vi "Thermocouple - SW-Timed Input.vi"() -> ()   [LabVIEW 2022 SP3]
doc: "This example demonstrates how to continuously acquire thermocouple measurements using a DAQmx device.\n\nFor instructions on how to connect your signals to the DAQ device, refer to your device documentation."
uses:
  <vilib>/Utility/error.llb/DialogType.ctl
  <vilib>/DAQmx/read.llb/DAQmx Read (Analog 1D Wfm NChan 1Samp).vi
  <vilib>/DAQmx/create/channels.llb/DAQmx Create Channel (AI-Temperature-Thermocouple).vi
  <vilib>/DAQmx/miscellaneous.llb/DAQmx Fill In Error Info.vi
  <resource>/objmgr/daqmx.rc
panel:
  in  "Auto Zero Mode":i32(ring)=10230 items=["None"=10230, "Once"=10244, "Every Sample"=10164]
  in  "CJC Channel":refnum<k21>
  in  "CJC Value":dbl=25.0 format="%0.2f"
  in  "CJC Source":i32(ring)=10116 items=["Built-In"=10200, "Constant Value"=10116, "Channel"=10113]
  in  "Thermocouple Type":i32(ring)=10072 items=["J"=10072, "K"=10073, "N"=10077, "R"=10082, "S"=10085, "T"=10086, "B"=10047, "E"=10055]
  in  "Units":i32(ring)=10143 items=["Deg C"=10143, "Deg F"=10144, "Kelvins"=10325, "Deg R"=10145, "From Custom Scale"=10065]
  in  "Loop Time (ms)":u32=100
  in  "Stop":bool
  in  "Max Temperature":dbl=100.0
  in  "Min Temperature":dbl
  in  "Physical Channel":tag="Dev1/ai0"
  out "Waveform Chart":waveform(dbl)[](graph)
  # "Acquired Data"
  # "Channel Settings"
  # "Timing Settings"
  # "Auto Zero Settings"
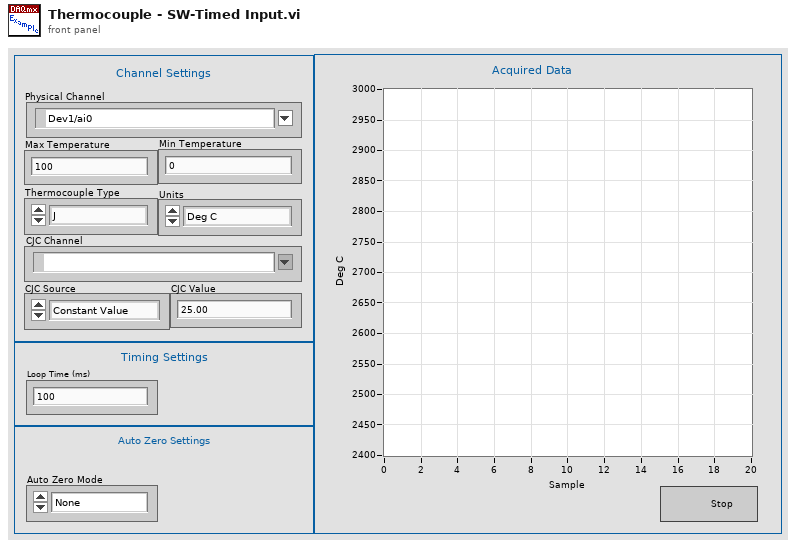
[diagram p1: front panel]
types:
  T1 = typedef "DialogType.ctl" = u16
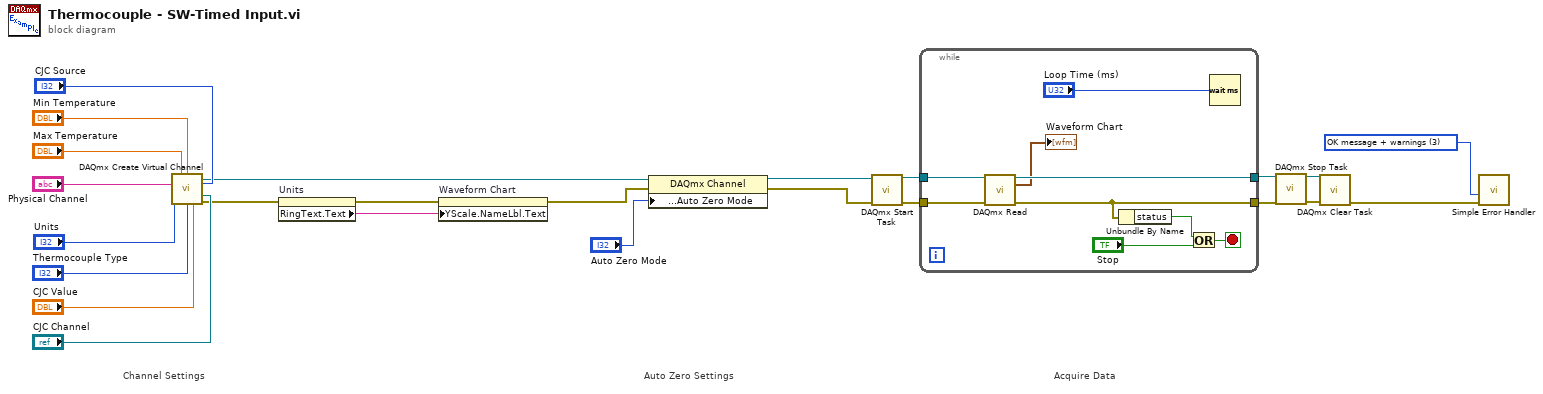
[diagram p0: block diagram]
diagram:
  w1 = T1 3 items=["no dialog", "OK message", "continue or stop message", "OK message + warnings", "continue/stop + warnings"] ("type of dialog (OK msg:1)")
  # "Auto Zero Settings"
  # "Acquire Data"
  # "Channel Settings"
  n1 = call-poly <vilib>:"DAQmx Create Virtual Channel.vi"("maximum value"="Max Temperature", "minimum value"="Min Temperature", "physical channels"="Physical Channel", "cjc source"="CJC Source", "units"="Units", "cjc channel"="CJC Channel", "thermocouple type"="Thermocouple Type", "cjc value"="CJC Value") -> ("task out"=w11:refnum<k21>, "error out"=w13:errorcluster)  [unwired: 6 in]
  n2 = property on="Units" class="Ring (strict)"(error in=w13) -> (error out=w7:errorcluster, "RingText.Text"=w8:string)  [unwired: 1 in, 1 out]
  n3 = property on="Waveform Chart" class="WFChart (strict)"(error in=w7, "YScale.NameLbl.Text"=w8) -> (error out=w6:errorcluster)  [unwired: 1 in, 1 out]
  n4 = property class="DAQmx Channel"(reference=w11, error in=w6, "Analog Input:General Properties:Advanced:High Accuracy Settings:Auto Zero Mode"="Auto Zero Mode") -> (reference out=w10:refnum<k21>, error out=w9:errorcluster)
  n5 = call <vilib>:"DAQmx Start Task.vi"("task/channels in"=w10, "error in"=w9) -> ("task out"=w24:refnum<k21>, "error out"=w23:errorcluster)  [unwired: 12 in]
  n6 = while {
    tunnel: w24 -> [w33]
    tunnel: w23 -> [w32]
    tunnel: [w29] -> w2
    tunnel: [w30] -> w3
    stop <- w31 stop-if-true
    n7 = call-poly <vilib>:"DAQmx Read.vi"("task/channels in"=w33, "error in"=w32) -> ("task out"=w30:refnum<k21>, "data"=→"Waveform Chart":waveform(dbl)[], "error out"=w29:errorcluster)  [unwired: 11 in]
    n8 = Unbundle By Name(w29) -> ("status"=w28:bool)
    n9 = Or(x=w28, y="Stop") -> (x .or. y?=w31:bool)
    n10 = Wait (ms)(milliseconds to wait="Loop Time (ms)") -> ()  [unwired: 1 out]
  }
  n11 = call <vilib>:"DAQmx Stop Task.vi"("task/channels in"=w3, "error in"=w2) -> ("task out"=w5:refnum<k21>, "error out"=w4:errorcluster)  [unwired: 12 in]
  n12 = call <vilib>:"DAQmx Clear Task.vi"("task in"=w5, "error in"=w4) -> ("error out"=w22:errorcluster)  [unwired: 13 in]
  n13 = call <vilib>:"Simple Error Handler.vi"("type of dialog (OK msg:1)"=w1, "error in (no error)"=w22) -> ()  [unwired: 3 in, 5 out]
